vi "FipsAdjacent.vi"() -> (11 "Fips":i32[](array[numeric]))   [LabVIEW 2017] (continued)
\"Posey County, IN\"\t18129\n\"Posey County, IN\"\t18129\t\"Vanderburgh County, IN\"\t18163\n\"Posey County, IN\"\t18129\t\"Henderson County, KY\"\t21101\n\"Posey County, IN\"\t18129\t\"Union County, KY\"\t21225\n\"Pulaski County, IN\"\t18131\t\"Cass County, IN\"\t18017\n\"Pulaski County, IN\"\t18131\t\"Fulton County, IN\"\t18049\n\"Pulaski County, IN\"\t18131\t\"Jasper County, IN\"\t18073\n\"Pulaski County, IN\"\t18131\t\"Marshall County, IN\"\t18099\n\"Pulaski County, IN\"\t18131\t\"Pulaski County, IN\"\t18131\n\"Pulaski County, IN\"\t18131\t\"Starke County, IN\"\t18149\n\"Pulaski County, IN\"\t18131\t\"White County, IN\"\t18181\n\"Putnam County, IN\"\t18133\t\"Clay County, IN\"\t18021\n\"Putnam County, IN\"\t18133\t\"Hendricks County, IN\"\t18063\n\"Putnam County, IN\"\t18133\t\"Montgomery County, IN\"\t18107\n\"Putnam County, IN\"\t18133\t\"Morgan County, IN\"\t18109\n\"Putnam County, IN\"\t18133\t\"Owen County, IN\"\t18119\n\"Putnam County, IN\"\t18133\t\"Parke County, IN\"\t18121\n\"Putnam County, IN\"\t18133\t\"Putnam County, IN\"\t18133\n\"Randolph County, IN\"\t18135\t\"Delaware County, IN\"\t18035\n\"Randolph County, IN\"\t18135\t\"Henry County, IN\"\t18065\n\"Randolph County, IN\"\t18135\t\"Jay County, IN\"\t18075\n\"Randolph County, IN\"\t18135\t\"Randolph County, IN\"\t18135\n\"Randolph County, IN\"\t18135\t\"Wayne County, IN\"\t18177\n\"Randolph County, IN\"\t18135\t\"Darke County, OH\"\t39037\n\"Ripley County, IN\"\t18137\t\"Dearborn County, IN\"\t18029\n\"Ripley County, IN\"\t18137\t\"Decatur County, IN\"\t18031\n\"Ripley County, IN\"\t18137\t\"Franklin County, IN\"\t18047\n\"Ripley County, IN\"\t18137\t\"Jefferson County, IN\"\t18077\n\"Ripley County, IN\"\t18137\t\"Jennings County, IN\"\t18079\n\"Ripley County, IN\"\t18137\t\"Ohio County, IN\"\t18115\n\"Ripley County, IN\"\t18137\t\"Ripley County, IN\"\t18137\n\"Ripley County, IN\"\t18137\t\"Switzerland County, IN\"\t18155\n\"Rush County, IN\"\t18139\t\"Decatur County, IN\"\t18031\n\"Rush County, IN\"\t18139\t\"Fayette County, IN\"\t18041\n\"Rush County, IN\"\t18139\t\"Franklin County, IN\"\t18047\n\"Rush County, IN\"\t18139\t\"Hancock County, IN\"\t18059\n\"Rush County, IN\"\t18139\t\"Henry County, IN\"\t18065\n\"Rush County, IN\"\t18139\t\"Rush County, IN\"\t18139\n\"Rush County, IN\"\t18139\t\"Shelby County, IN\"\t18145\n\"St. Joseph County, IN\"\t18141\t\"Elkhart County, IN\"\t18039\n\"St. Joseph County, IN\"\t18141\t\"LaPorte County, IN\"\t18091\n\"St. Joseph County, IN\"\t18141\t\"Marshall County, IN\"\t18099\n\"St. Joseph County, IN\"\t18141\t\"St. Joseph County, IN\"\t18141\n\"St. Joseph County, IN\"\t18141\t\"Starke County, IN\"\t18149\n\"St. Joseph County, IN\"\t18141\t\"Berrien County, MI\"\t26021\n\"St. Joseph County, IN\"\t18141\t\"Cass County, MI\"\t26027\n\"Scott County, IN\"\t18143\t\"Clark County, IN\"\t18019\n\"Scott County, IN\"\t18143\t\"Jackson County, IN\"\t18071\n\"Scott County, IN\"\t18143\t\"Jefferson County, IN\"\t18077\n\"Scott County, IN\"\t18143\t\"Jennings County, IN\"\t18079\n\"Scott County, IN\"\t18143\t\"Scott County, IN\"\t18143\n\"Scott County, IN\"\t18143\t\"Washington County, IN\"\t18175\n\"Shelby County, IN\"\t18145\t\"Bartholomew County, IN\"\t18005\n\"Shelby County, IN\"\t18145\t\"Decatur County, IN\"\t18031\n\"Shelby County, IN\"\t18145\t\"Hancock County, IN\"\t18059\n\"Shelby County, IN\"\t18145\t\"Johnson County, IN\"\t18081\n\"Shelby County, IN\"\t18145\t\"Marion County, IN\"\t18097\n\"Shelby County, IN\"\t18145\t\"Rush County, IN\"\t18139\n\"Shelby County, IN\"\t18145\t\"Shelby County, IN\"\t18145\n\"Spencer County, IN\"\t18147\t\"Dubois County, IN\"\t18037\n\"Spencer County, IN\"\t18147\t\"Perry County, IN\"\t18123\n\"Spencer County, IN\"\t18147\t\"Spencer County, IN\"\t18147\n\"Spencer County, IN\"\t18147\t\"Warrick County, IN\"\t18173\n\"Spencer County, IN\"\t18147\t\"Daviess County, KY\"\t21059\n\"Spencer County, IN\"\t18147\t\"Hancock County, KY\"\t21091\n\"Starke County, IN\"\t18149\t\"Fulton County, IN\"\t18049\n\"Starke County, IN\"\t18149\t\"Jasper County, IN\"\t18073\n\"Starke County, IN\"\t18149\t\"LaPorte County, IN\"\t18091\n\"Starke County, IN\"\t18149\t\"Marshall County, IN\"\t18099\n\"Starke County, IN\"\t18149\t\"Porter County, IN\"\t18127\n\"Starke County, IN\"\t18149\t\"Pulaski County, IN\"\t18131\n\"Starke County, IN\"\t18149\t\"St. Joseph County, IN\"\t18141\n\"Starke County, IN\"\t18149\t\"Starke County, IN\"\t18149\n\"Steuben County, IN\"\t18151\t\"DeKalb County, IN\"\t18033\n\"Steuben County, IN\"\t18151\t\"LaGrange County, IN\"\t18087\n\"Steuben County, IN\"\t18151\t\"Noble County, IN\"\t18113\n\"Steuben County, IN\"\t18151\t\"Steuben County, IN\"\t18151\n\"Steuben County, IN\"\t18151\t\"Branch County, MI\"\t26023\n\"Steuben County, IN\"\t18151\t\"Hillsdale County, MI\"\t26059\n\"Steuben County, IN\"\t18151\t\"Williams County, OH\"\t39171\n\"Sullivan County, IN\"\t18153\t\"Clark County, IL\"\t17023\n\"Sullivan County, IN\"\t18153\t\"Crawford County, IL\"\t17033\n\"Sullivan County, IN\"\t18153\t\"Clay County, IN\"\t18021\n\"Sullivan County, IN\"\t18153\t\"Greene County, IN\"\t18055\n\"Sullivan County, IN\"\t18153\t\"Knox County, IN\"\t18083\n\"Sullivan County, IN\"\t18153\t\"Sullivan County, IN\"\t18153\n\"Sullivan County, IN\"\t18153\t\"Vigo County, IN\"\t18167\n\"Switzerland County, IN\"\t18155\t\"Jefferson County, IN\"\t18077\n\"Switzerland County, IN\"\t18155\t\"Ohio County, IN\"\t18115\n\"Switzerland County, IN\"\t18155\t\"Ripley County, IN\"\t18137\n\"Switzerland County, IN\"\t18155\t\"Switzerland County, IN\"\t18155\n\"Switzerland County, IN\"\t18155\t\"Boone County, KY\"\t21015\n\"Switzerland County, IN\"\t18155\t\"Carroll County, KY\"\t21041\n\"Switzerland County, IN\"\t18155\t\"Gallatin County, KY\"\t21077\n\"Tippecanoe County, IN\"\t18157\t\"Benton County, IN\"\t18007\n\"Tippecanoe County, IN\"\t18157\t\"Carroll County, IN\"\t18015\n\"Tippecanoe County, IN\"\t18157\t\"Clinton County, IN\"\t18023\n\"Tippecanoe County, IN\"\t18157\t\"Fountain County, IN\"\t18045\n\"Tippecanoe County, IN\"\t18157\t\"Montgomery County, IN\"\t18107\n\"Tippecanoe County, IN\"\t18157\t\"Tippecanoe County, IN\"\t18157\n\"Tippecanoe County, IN\"\t18157\t\"Warren County, IN\"\t18171\n\"Tippecanoe County, IN\"\t18157\t\"White County, IN\"\t18181\n\"Tipton County, IN\"\t18159\t\"Clinton County, IN\"\t18023\n\"Tipton County, IN\"\t18159\t\"Grant County, IN\"\t18053\n\"Tipton County, IN\"\t18159\t\"Hamilton County, IN\"\t18057\n\"Tipton County, IN\"\t18159\t\"Howard County, IN\"\t18067\n\"Tipton County, IN\"\t18159\t\"Madison County, IN\"\t18095\n\"Tipton County, IN\"\t18159\t\"Tipton County, IN\"\t18159\n\"Union County, IN\"\t18161\t\"Fayette County, IN\"\t18041\n\"Union County, IN\"\t18161\t\"Franklin County, IN\"\t18047\n\"Union County, IN\"\t18161\t\"Union County, IN\"\t18161\n\"Union County, IN\"\t18161\t\"Wayne County, IN\"\t18177\n\"Union County, IN\"\t18161\t\"Butler County, OH\"\t39017\n\"Union County, IN\"\t18161\t\"Preble County, OH\"\t39135\n\"Vanderburgh County, IN\"\t18163\t\"Gibson County, IN\"\t18051\n\"Vanderburgh County, IN\"\t18163\t\"Posey County, IN\"\t18129\n\"Vanderburgh County, IN\"\t18163\t\"Vanderburgh County, IN\"\t18163\n\"Vanderburgh County, IN\"\t18163\t\"Warrick County, IN\"\t18173\n\"Vanderburgh County, IN\"\t18163\t\"Henderson County, KY\"\t21101\n\"Vermillion County, IN\"\t18165\t\"Edgar County, IL\"\t17045\n\"Vermillion County, IN\"\t18165\t\"Vermilion County, IL\"\t17183\n\"Vermillion County, IN\"\t18165\t\"Fountain County, IN\"\t18045\n\"Vermillion County, IN\"\t18165\t\"Parke County, IN\"\t18121\n\"Vermillion County, IN\"\t18165\t\"Vermillion County, IN\"\t18165\n\"Vermillion County, IN\"\t18165\t\"Vigo County, IN\"\t18167\n\"Vermillion County, IN\"\t18165\t\"Warren County, IN\"\t18171\n\"Vigo County, IN\"\t18167\t\"Clark County, IL\"\t17023\n\"Vigo County, IN\"\t18167\t\"Edgar County, IL\"\t17045\n\"Vigo County, IN\"\t18167\t\"Clay County, IN\"\t18021\n\"Vigo County, IN\"\t18167\t\"Parke County, IN\"\t18121\n\"Vigo County, IN\"\t18167\t\"Sullivan County, IN\"\t18153\n\"Vigo County, IN\"\t18167\t\"Vermillion County, IN\"\t18165\n\"Vigo County, IN\"\t18167\t\"Vigo County, IN\"\t18167\n\"Wabash County, IN\"\t18169\t\"Fulton County, IN\"\t18049\n\"Wabash County, IN\"\t18169\t\"Grant County, IN\"\t18053\n\"Wabash County, IN\"\t18169\t\"Huntington County, IN\"\t18069\n\"Wabash County, IN\"\t18169\t\"Kosciusko County, IN\"\t18085\n\"Wabash County, IN\"\t18169\t\"Miami County, IN\"\t18103\n\"Wabash County, IN\"\t18169\t\"Wabash County, IN\"\t18169\n\"Wabash County, IN\"\t18169\t\"Whitley County, IN\"\t18183\n\"Warren County, IN\"\t18171\t\"Vermilion County, IL\"\t17183\n\"Warren County, IN\"\t18171\t\"Benton County, IN\"\t18007\n\"Warren County, IN\"\t18171\t\"Fountain County, IN\"\t18045\n\"Warren County, IN\"\t18171\t\"Tippecanoe County, IN\"\t18157\n\"Warren County, IN\"\t18171\t\"Vermillion County, IN\"\t18165\n\"Warren County, IN\"\t18171\t\"Warren County, IN\"\t18171\n\"Warrick County, IN\"\t18173\t\"Dubois County, IN\"\t18037\n\"Warrick County, IN\"\t18173\t\"Gibson County, IN\"\t18051\n\"Warrick County, IN\"\t18173\t\"Pike County, IN\"\t18125\n\"Warrick County, IN\"\t18173\t\"Spencer County, IN\"\t18147\n\"Warrick County, IN\"\t18173\t\"Vanderburgh County, IN\"\t18163\n\"Warrick County, IN\"\t18173\t\"Warrick County, IN\"\t18173\n\"Warrick County, IN\"\t18173\t\"Daviess County, KY\"\t21059\n\"Warrick County, IN\"\t18173\t\"Henderson County, KY\"\t21101\n\"Washington County, IN\"\t18175\t\"Clark County, IN\"\t18019\n\"Washington County, IN\"\t18175\t\"Crawford County, IN\"\t18025\n\"Washington County, IN\"\t18175\t\"Floyd County, IN\"\t18043\n\"Washington County, IN\"\t18175\t\"Harrison County, IN\"\t18061\n\"Washington County, IN\"\t18175\t\"Jackson County, IN\"\t18071\n\"Washington County, IN\"\t18175\t\"Lawrence County, IN\"\t18093\n\"Washington County, IN\"\t18175\t\"Orange County, IN\"\t18117\n\"Washington County, IN\"\t18175\t\"Scott County, IN\"\t18143\n\"Washington County, IN\"\t18175\t\"Washington County, IN\"\t18175\n\"Wayne County, IN\"\t18177\t\"Fayette County, IN\"\t18041\n\"Wayne County, IN\"\t18177\t\"Henry County, IN\"\t18065\n\"Wayne County, IN\"\t18177\t\"Randolph County, IN\"\t18135\n\"Wayne County, IN\"\t18177\t\"Union County, IN\"\t18161\n\"Wayne County, IN\"\t18177\t\"Wayne County, IN\"\t18177\n\"Wayne County, IN\"\t18177\t\"Darke County, OH\"\t39037\n\"Wayne County, IN\"\t18177\t\"Preble County, OH\"\t39135\n\"Wells County, IN\"\t18179\t\"Adams County, IN\"\t18001\n\"Wells County, IN\"\t18179\t\"Allen County, IN\"\t18003\n\"Wells County, IN\"\t18179\t\"Blackford County, IN\"\t18009\n\"Wells County, IN\"\t18179\t\"Grant County, IN\"\t18053\n\"Wells County, IN\"\t18179\t\"Huntington County, IN\"\t18069\n\"Wells County, IN\"\t18179\t\"Jay County, IN\"\t18075\n\"Wells County, IN\"\t18179\t\"Wells County, IN\"\t18179\n\"White County, IN\"\t18181\t\"Benton County, IN\"\t18007\n\"White County, IN\"\t18181\t\"Carroll County, IN\"\t18015\n\"White County, IN\"\t18181\t\"Cass County, IN\"\t18017\n\"White County, IN\"\t18181\t\"Jasper County, IN\"\t18073\n\"White County, IN\"\t18181\t\"Pulaski County, IN\"\t18131\n\"White County, IN\"\t18181\t\"Tippecanoe County, IN\"\t18157\n\"White County, IN\"\t18181\t\"White County, IN\"\t18181\n\"Whitley County, IN\"\t18183\t\"Allen County, IN\"\t18003\n\"Whitley County, IN\"\t18183\t\"Huntington County, IN\"\t18069\n\"Whitley County, IN\"\t18183\t\"Kosciusko County, IN\"\t18085\n\"Whitley County, IN\"\t18183\t\"Noble County, IN\"\t18113\n\"Whitley County, IN\"\t18183\t\"Wabash County, IN\"\t18169\n\"Whitley County, IN\"\t18183\t\"Whitley County, IN\"\t18183\n\"Adair County, IA\"\t19001\t\"Adair County, IA\"\t19001\n\"Adair County, IA\"\t19001\t\"Adams County, IA\"\t19003\n\"Adair County, IA\"\t19001\t\"Audubon County, IA\"\t19009\n\"Adair County, IA\"\t19001\t\"Cass County, IA\"\t19029\n\"Adair County, IA\"\t19001\t\"Dallas County, IA\"\t19049\n\"Adair County, IA\"\t19001\t\"Guthrie County, IA\"\t19077\n\"Adair County, IA\"\t19001\t\"Madison County, IA\"\t19121\n\"Adair County, IA\"\t19001\t\"Union County, IA\"\t19175\n\"Adams County, IA\"\t19003\t\"Adair County, IA\"\t19001\n\"Adams County, IA\"\t19003\t\"Adams County, IA\"\t19003\n\"Adams County, IA\"\t19003\t\"Cass County, IA\"\t19029\n\"Adams County, IA\"\t19003\t\"Montgomery County, IA\"\t19137\n\"Adams County, IA\"\t19003\t\"Page County, IA\"\t19145\n\"Adams County, IA\"\t19003\t\"Ringgold County, IA\"\t19159\n\"Adams County, IA\"\t19003\t\"Taylor County, IA\"\t19173\n\"Adams County, IA\"\t19003\t\"Union County, IA\"\t19175\n\"Allamakee County, IA\"\t19005\t\"Allamakee County, IA\"\t19005\n\"Allamakee County, IA\"\t19005\t\"Clayton County, IA\"\t19043\n\"Allamakee County, IA\"\t19005\t\"Fayette County, IA\"\t19065\n\"Allamakee County, IA\"\t19005\t\"Winneshiek County, IA\"\t19191\n\"Allamakee County, IA\"\t19005\t\"Houston County, MN\"\t27055\n\"Allamakee County, IA\"\t19005\t\"Crawford County, WI\"\t55023\n\"Allamakee County, IA\"\t19005\t\"Vernon County, WI\"\t55123\n\"Appanoose County, IA\"\t19007\t\"Appanoose County, IA\"\t19007\n\"Appanoose County, IA\"\t19007\t\"Davis County, IA\"\t19051\n\"Appanoose County, IA\"\t19007\t\"Lucas County, IA\"\t19117\n\"Appanoose County, IA\"\t19007\t\"Monroe County, IA\"\t19135\n\"Appanoose County, IA\"\t19007\t\"Wapello County, IA\"\t19179\n\"Appanoose County, IA\"\t19007\t\"Wayne County, IA\"\t19185\n\"Appanoose County, IA\"\t19007\t\"Putnam County, MO\"\t29171\n\"Appanoose County, IA\"\t19007\t\"Schuyler County, MO\"\t29197\n\"Audubon County, IA\"\t19009\t\"Adair County, IA\"\t19001\n\"Audubon County, IA\"\t19009\t\"Audubon County, IA\"\t19009\n\"Audubon County, IA\"\t19009\t\"Carroll County, IA\"\t19027\n\"Audubon County, IA\"\t19009\t\"Cass County, IA\"\t19029\n\"Audubon County, IA\"\t19009\t\"Crawford County, IA\"\t19047\n\"Audubon County, IA\"\t19009\t\"Guthrie County, IA\"\t19077\n\"Audubon County, IA\"\t19009\t\"Shelby County, IA\"\t19165\n\"Benton County, IA\"\t19011\t\"Benton County, IA\"\t19011\n\"Benton County, IA\"\t19011\t\"Black Hawk County, IA\"\t19013\n\"Benton County, IA\"\t19011\t\"Buchanan County, IA\"\t19019\n\"Benton County, IA\"\t19011\t\"Iowa County, IA\"\t19095\n\"Benton County, IA\"\t19011\t\"Johnson County, IA\"\t19103\n\"Benton County, IA\"\t19011\t\"Linn County, IA\"\t19113\n\"Benton County, IA\"\t19011\t\"Poweshiek County, IA\"\t19157\n\"Benton County, IA\"\t19011\t\"Tama County, IA\"\t19171\n\"Black Hawk County, IA\"\t19013\t\"Benton County, IA\"\t19011\n\"Black Hawk County, IA\"\t19013\t\"Black Hawk County, IA\"\t19013\n\"Black Hawk County, IA\"\t19013\t\"Bremer County, IA\"\t19017\n\"Black Hawk County, IA\"\t19013\t\"Buchanan County, IA\"\t19019\n\"Black Hawk County, IA\"\t19013\t\"Butler County, IA\"\t19023\n\"Black Hawk County, IA\"\t19013\t\"Fayette County, IA\"\t19065\n\"Black Hawk County, IA\"\t19013\t\"Grundy County, IA\"\t19075\n\"Black Hawk County, IA\"\t19013\t\"Tama County, IA\"\t19171\n\"Boone County, IA\"\t19015\t\"Boone County, IA\"\t19015\n\"Boone County, IA\"\t19015\t\"Dallas County, IA\"\t19049\n\"Boone County, IA\"\t19015\t\"Greene County, IA\"\t19073\n\"Boone County, IA\"\t19015\t\"Hamilton County, IA\"\t19079\n\"Boone County, IA\"\t19015\t\"Polk County, IA\"\t19153\n\"Boone County, IA\"\t19015\t\"Story County, IA\"\t19169\n\"Boone County, IA\"\t19015\t\"Webster County, IA\"\t19187\n\"Bremer County, IA\"\t19017\t\"Black Hawk County, IA\"\t19013\n\"Bremer County, IA\"\t19017\t\"Bremer County, IA\"\t19017\n\"Bremer County, IA\"\t19017\t\"Buchanan County, IA\"\t19019\n\"Bremer County, IA\"\t19017\t\"Butler County, IA\"\t19023\n\"Bremer County, IA\"\t19017\t\"Chickasaw County, IA\"\t19037\n\"Bremer County, IA\"\t19017\t\"Fayette County, IA\"\t19065\n\"Bremer County, IA\"\t19017\t\"Floyd County, IA\"\t19067\n\"Buchanan County, IA\"\t19019\t\"Benton County, IA\"\t19011\n\"Buchanan County, IA\"\t19019\t\"Black Hawk County, IA\"\t19013\n\"Buchanan County, IA\"\t19019\t\"Bremer County, IA\"\t19017\n\"Buchanan County, IA\"\t19019\t\"Buchanan County, IA\"\t19019\n\"Buchanan County, IA\"\t19019\t\"Clayton County, IA\"\t19043\n\"Buchanan County, IA\"\t19019\t\"Delaware County, IA\"\t19055\n\"Buchanan County, IA\"\t19019\t\"Fayette County, IA\"\t19065\n\"Buchanan County, IA\"\t19019\t\"Linn County, IA\"\t19113\n\"Buena Vista County, IA\"\t19021\t\"Buena Vista County, IA\"\t19021\n\"Buena Vista County, IA\"\t19021\t\"Calhoun County, IA\"\t19025\n\"Buena Vista County, IA\"\t19021\t\"Cherokee County, IA\"\t19035\n\"Buena Vista County, IA\"\t19021\t\"Clay County, IA\"\t19041\n\"Buena Vista County, IA\"\t19021\t\"Ida County, IA\"\t19093\n\"Buena Vista County, IA\"\t19021\t\"O'Brien County, IA\"\t19141\n\"Buena Vista County, IA\"\t19021\t\"Palo Alto County, IA\"\t19147\n\"Buena Vista County, IA\"\t19021\t\"Pocahontas County, IA\"\t19151\n\"Buena Vista County, IA\"\t19021\t\"Sac County, IA\"\t19161\n\"Butler County, IA\"\t19023\t\"Black Hawk County, IA\"\t19013\n\"Butler County, IA\"\t19023\t\"Bremer County, IA\"\t19017\n\"Butler County, IA\"\t19023\t\"Butler County, IA\"\t19023\n\"Butler County, IA\"\t19023\t\"Cerro Gordo County, IA\"\t19033\n\"Butler County, IA\"\t19023\t\"Chickasaw County, IA\"\t19037\n\"Butler County, IA\"\t19023\t\"Floyd County, IA\"\t19067\n\"Butler County, IA\"\t19023\t\"Franklin County, IA\"\t19069\n\"Butler County, IA\"\t19023\t\"Grundy County, IA\"\t19075\n\"Butler County, IA\"\t19023\t\"Hardin County, IA\"\t19083\n\"Calhoun County, IA\"\t19025\t\"Buena Vista County, IA\"\t19021\n\"Calhoun County, IA\"\t19025\t\"Calhoun County, IA\"\t19025\n\"Calhoun County, IA\"\t19025\t\"Carroll County, IA\"\t19027\n\"Calhoun County, IA\"\t19025\t\"Greene County, IA\"\t19073\n\"Calhoun County, IA\"\t19025\t\"Pocahontas County, IA\"\t19151\n\"Calhoun County, IA\"\t19025\t\"Sac County, IA\"\t19161\n\"Calhoun County, IA\"\t19025\t\"Webster County, IA\"\t19187\n\"Carroll County, IA\"\t19027\t\"Audubon County, IA\"\t19009\n\"Carroll County, IA\"\t19027\t\"Calhoun County, IA\"\t19025\n\"Carroll County, IA\"\t19027\t\"Carroll County, IA\"\t19027\n\"Carroll County, IA\"\t19027\t\"Crawford County, IA\"\t19047\n\"Carroll County, IA\"\t19027\t\"Greene County, IA\"\t19073\n\"Carroll County, IA\"\t19027\t\"Guthrie County, IA\"\t19077\n\"Carroll County, IA\"\t19027\t\"Sac County, IA\"\t19161\n\"Carroll County, IA\"\t19027\t\"Shelby County, IA\"\t19165\n\"Cass County, IA\"\t19029\t\"Adair County, IA\"\t19001\n\"Cass County, IA\"\t19029\t\"Adams County, IA\"\t19003\n\"Cass County, IA\"\t19029\t\"Audubon County, IA\"\t19009\n\"Cass County, IA\"\t19029\t\"Cass County, IA\"\t19029\n\"Cass County, IA\"\t19029\t\"Guthrie County, IA\"\t19077\n\"Cass County, IA\"\t19029\t\"Montgomery County, IA\"\t19137\n\"Cass County, IA\"\t19029\t\"Pottawattamie County, IA\"\t19155\n\"Cass County, IA\"\t19029\t\"Shelby County, IA\"\t19165\n\"Cedar County, IA\"\t19031\t\"Cedar County, IA\"\t19031\n\"Cedar County, IA\"\t19031\t\"Clinton County, IA\"\t19045\n\"Cedar County, IA\"\t19031\t\"Johnson County, IA\"\t19103\n\"Cedar County, IA\"\t19031\t\"Jones County, IA\"\t19105\n\"Cedar County, IA\"\t19031\t\"Linn County, IA\"\t19113\n\"Cedar County, IA\"\t19031\t\"Muscatine County, IA\"\t19139\n\"Cedar County, IA\"\t19031\t\"Scott County, IA\"\t19163\n\"Cerro Gordo County, IA\"\t19033\t\"Butler County, IA\"\t19023\n\"Cerro Gordo County, IA\"\t19033\t\"Cerro Gordo County, IA\"\t19033\n\"Cerro Gordo County, IA\"\t19033\t\"Floyd County, IA\"\t19067\n\"Cerro Gordo County, IA\"\t19033\t\"Franklin County, IA\"\t19069\n\"Cerro Gordo County, IA\"\t19033\t\"Hancock County, IA\"\t19081\n\"Cerro Gordo County, IA\"\t19033\t\"Mitchell County, IA\"\t19131\n\"Cerro Gordo County, IA\"\t19033\t\"Winnebago County, IA\"\t19189\n\"Cerro Gordo County, IA\"\t19033\t\"Worth County, IA\"\t19195\n\"Cerro Gordo County, IA\"\t19033\t\"Wright County, IA\"\t19197\n\"Cherokee County, IA\"\t19035\t\"Buena Vista County, IA\"\t19021\n\"Cherokee County, IA\"\t19035\t\"Cherokee County, IA\"\t19035\n\"Cherokee County, IA\"\t19035\t\"Clay County, IA\"\t19041\n\"Cherokee County, IA\"\t19035\t\"Ida County, IA\"\t19093\n\"Cherokee County, IA\"\t19035\t\"O'Brien County, IA\"\t19141\n\"Cherokee County, IA\"\t19035\t\"Plymouth County, IA\"\t19149\n\"Cherokee County, IA\"\t19035\t\"Sac County, IA\"\t19161\n\"Cherokee County, IA\"\t19035\t\"Sioux County, IA\"\t19167\n\"Cherokee County, IA\"\t19035\t\"Woodbury County, IA\"\t19193\n\"Chickasaw County, IA\"\t19037\t\"Bremer County, IA\"\t19017\n\"Chickasaw County, IA\"\t19037\t\"Butler County, IA\"\t19023\n\"Chickasaw County, IA\"\t19037\t\"Chickasaw County, IA\"\t19037\n\"Chickasaw County, IA\"\t19037\t\"Fayette County, IA\"\t19065\n\"Chickasaw County, IA\"\t19037\t\"Floyd County, IA\"\t19067\n\"Chickasaw County, IA\"\t19037\t\"Howard County, IA\"\t19089\n\"Chickasaw County, IA\"\t19037\t\"Mitchell County, IA\"\t19131\n\"Chickasaw County, IA\"\t19037\t\"Winneshiek County, IA\"\t19191\n\"Clarke County, IA\"\t19039\t\"Clarke County, IA\"\t19039\n\"Clarke County, IA\"\t19039\t\"Decatur County, IA\"\t19053\n\"Clarke County, IA\"\t19039\t\"Lucas County, IA\"\t19117\n\"Clarke County, IA\"\t19039\t\"Madison County, IA\"\t19121\n\"Clarke County, IA\"\t19039\t\"Ringgold County, IA\"\t19159\n\"Clarke County, IA\"\t19039\t\"Union County, IA\"\t19175\n\"Clarke County, IA\"\t19039\t\"Warren County, IA\"\t19181\n\"Clarke County, IA\"\t19039\t\"Wayne County, IA\"\t19185\n\"Clay County, IA\"\t19041\t\"Buena Vista County, IA\"\t19021\n\"Clay County, IA\"\t19041\t\"Cherokee County, IA\"\t19035\n\"Clay County, IA\"\t19041\t\"Clay County, IA\"\t19041\n\"Clay County, IA\"\t19041\t\"Dickinson County, IA\"\t19059\n\"Clay County, IA\"\t19041\t\"Emmet County, IA\"\t19063\n\"Clay County, IA\"\t19041\t\"O'Brien County, IA\"\t19141\n\"Clay County, IA\"\t19041\t\"Osceola County, IA\"\t19143\n\"Clay County, IA\"\t19041\t\"Palo Alto County, IA\"\t19147\n\"Clay County, IA\"\t19041\t\"Pocahontas County, IA\"\t19151\n\"Clayton County, IA\"\t19043\t\"Allamakee County, IA\"\t19005\n\"Clayton County, IA\"\t19043\t\"Buchanan County, IA\"\t19019\n\"Clayton County, IA\"\t19043\t\"Clayton County, IA\"\t19043\n\"Clayton County, IA\"\t19043\t\"Delaware County, IA\"\t19055\n\"Clayton County, IA\"\t19043\t\"Dubuque County, IA\"\t19061\n\"Clayton County, IA\"\t19043\t\"Fayette County, IA\"\t19065\n\"Clayton County, IA\"\t19043\t\"Winneshiek County, IA\"\t19191\n\"Clayton County, IA\"\t19043\t\"Crawford County, WI\"\t55023\n\"Clayton County, IA\"\t19043\t\"Grant County, WI\"\t55043\n\"Clinton County, IA\"\t19045\t\"Carroll County, IL\"\t17015\n\"Clinton County, IA\"\t19045\t\"Rock Island County, IL\"\t17161\n\"Clinton County, IA\"\t19045\t\"Whiteside County, IL\"\t17195\n\"Clinton County, IA\"\t19045\t\"Cedar County, IA\"\t19031\n\"Clinton County, IA\"\t19045\t\"Clinton County, IA\"\t19045\n\"Clinton County, IA\"\t19045\t\"Jackson County, IA\"\t19097\n\"Clinton County, IA\"\t19045\t\"Jones County, IA\"\t19105\n\"Clinton County, IA\"\t19045\t\"Scott County, IA\"\t19163\n\"Crawford County, IA\"\t19047\t\"Audubon County, IA\"\t19009\n\"Crawford County, IA\"\t19047\t\"Carroll County, IA\"\t19027\n\"Crawford County, IA\"\t19047\t\"Crawford County, IA\"\t19047\n\"Crawford County, IA\"\t19047\t\"Harrison County, IA\"\t19085\n\"Crawford County, IA\"\t19047\t\"Ida County, IA\"\t19093\n\"Crawford County, IA\"\t19047\t\"Monona County, IA\"\t19133\n\"Crawford County, IA\"\t19047\t\"Sac County, IA\"\t19161\n\"Crawford County, IA\"\t19047\t\"Shelby County, IA\"\t19165\n\"Crawford County, IA\"\t19047\t\"Woodbury County, IA\"\t19193\n\"Dallas County, IA\"\t19049\t\"Adair County, IA\"\t19001\n\"Dallas County, IA\"\t19049\t\"Boone County, IA\"\t19015\n\"Dallas County, IA\"\t19049\t\"Dallas County, IA\"\t19049\n\"Dallas County, IA\"\t19049\t\"Greene County, IA\"\t19073\n\"Dallas County, IA\"\t19049\t\"Guthrie County, IA\"\t19077\n\"Dallas County, IA\"\t19049\t\"Madison County, IA\"\t19121\n\"Dallas County, IA\"\t19049\t\"Polk County, IA\"\t19153\n\"Dallas County, IA\"\t19049\t\"Warren County, IA\"\t19181\n\"Davis County, IA\"\t19051\t\"Appanoose County, IA\"\t19007\n\"Davis County, IA\"\t19051\t\"Davis County, IA\"\t19051\n\"Davis County, IA\"\t19051\t\"Jefferson County, IA\"\t19101\n\"Davis County, IA\"\t19051\t\"Monroe County, IA\"\t19135\n\"Davis County, IA\"\t19051\t\"Van Buren County, IA\"\t19177\n\"Davis County, IA\"\t19051\t\"Wapello County, IA\"\t19179\n\"Davis County, IA\"\t19051\t\"Schuyler County, MO\"\t29197\n\"Davis County, IA\"\t19051\t\"Scotland County, MO\"\t29199\n\"Decatur County, IA\"\t19053\t\"Clarke County, IA\"\t19039\n\"Decatur County, IA\"\t19053\t\"Decatur County, IA\"\t19053\n\"Decatur County, IA\"\t19053\t\"Lucas County, IA\"\t19117\n\"Decatur County, IA\"\t19053\t\"Ringgold County, IA\"\t19159\n\"Decatur County, IA\"\t19053\t\"Union County, IA\"\t19175\n\"Decatur County, IA\"\t19053\t\"Wayne County, IA\"\t19185\n\"Decatur County, IA\"\t19053\t\"Harrison County, MO\"\t29081\n\"Decatur County, IA\"\t19053\t\"Mercer County, MO\"\t29129\n\"Delaware County, IA\"\t19055\t\"Buchanan County, IA\"\t19019\n\"Delaware County, IA\"\t19055\t\"Clayton County, IA\"\t19043\n\"Delaware County, IA\"\t19055\t\"Delaware County, IA\"\t19055\n\"Delaware County, IA\"\t19055\t\"Dubuque County, IA\"\t19061\n\"Delaware County, IA\"\t19055\t\"Fayette County, IA\"\t19065\n\"Delaware County, IA\"\t19055\t\"Jones County, IA\"\t19105\n\"Delaware County, IA\"\t19055\t\"Linn County, IA\"\t19113\n\"Des Moines County, IA\"\t19057\t\"Henderson County, IL\"\t17071\n\"Des Moines County, IA\"\t19057\t\"Mercer County, IL\"\t17131\n\"Des Moines County, IA\"\t19057\t\"Des Moines County, IA\"\t19057\n\"Des Moines County, IA\"\t19057\t\"Henry County, IA\"\t19087\n\"Des Moines County, IA\"\t19057\t\"Lee County, IA\"\t19111\n\"Des Moines County, IA\"\t19057\t\"Louisa County, IA\"\t19115\n\"Dickinson County, IA\"\t19059\t\"Clay County, IA\"\t19041\n\"Dickinson County, IA\"\t19059\t\"Dickinson County, IA\"\t19059\n\"Dickinson County, IA\"\t19059\t\"Emmet County, IA\"\t19063\n\"Dickinson County, IA\"\t19059\t\"O'Brien County, IA\"\t19141\n\"Dickinson County, IA\"\t19059\t\"Osceola County, IA\"\t19143\n\"Dickinson County, IA\"\t19059\t\"Palo Alto County, IA\"\t19147\n\"Dickinson County, IA\"\t19059\t\"Jackson County, MN\"\t27063\n\"Dubuque County, IA\"\t19061\t\"Jo Daviess County, IL\"\t17085\n\"Dubuque County, IA\"\t19061\t\"Clayton County, IA\"\t19043\n\"Dubuque County, IA\"\t19061\t\"Delaware County, IA\"\t19055\n\"Dubuque County, IA\"\t19061\t\"Dubuque County, IA\"\t19061\n\"Dubuque County, IA\"\t19061\t\"Jackson County, IA\"\t19097\n\"Dubuque County, IA\"\t19061\t\"Jones County, IA\"\t19105\n\"Dubuque County, IA\"\t19061\t\"Grant County, WI\"\t55043\n\"Emmet County, IA\"\t19063\t\"Clay County, IA\"\t19041\n\"Emmet County, IA\"\t19063\t\"Dickinson County, IA\"\t19059\n\"Emmet County, IA\"\t19063\t\"Emmet County, IA\"\t19063\n\"Emmet County, IA\"\t19063\t\"Kossuth County, IA\"\t19109\n\"Emmet County, IA\"\t19063\t\"Palo Alto County, IA\"\t19147\n\"Emmet County, IA\"\t19063\t\"Jackson County, MN\"\t27063\n\"Emmet County, IA\"\t19063\t\"Martin County, MN\"\t27091\n\"Fayette County, IA\"\t19065\t\"Allamakee County, IA\"\t19005\n\"Fayette County, IA\"\t19065\t\"Black Hawk County, IA\"\t19013\n\"Fayette County, IA\"\t19065\t\"Bremer County, IA\"\t19017\n\"Fayette County, IA\"\t19065\t\"Buchanan County, IA\"\t19019\n\"Fayette County, IA\"\t19065\t\"Chickasaw County, IA\"\t19037\n\"Fayette County, IA\"\t19065\t\"Clayton County, IA\"\t19043\n\"Fayette County, IA\"\t19065\t\"Delaware County, IA\"\t19055\n\"Fayette County, IA\"\t19065\t\"Fayette County, IA\"\t19065\n\"Fayette County, IA\"\t19065\t\"Winneshiek County, IA\"\t19191\n\"Floyd County, IA\"\t19067\t\"Bremer County, IA\"\t19017\n\"Floyd County, IA\"\t19067\t\"Butler County, IA\"\t19023\n\"Floyd County, IA\"\t19067\t\"Cerro Gordo County, IA\"\t19033\n\"Floyd County, IA\"\t19067\t\"Chickasaw County, IA\"\t19037\n\"Floyd County, IA\"\t19067\t\"Floyd County, IA\"\t19067\n\"Floyd County, IA\"\t19067\t\"Franklin County, IA\"\t19069\n\"Floyd County, IA\"\t19067\t\"Howard County, IA\"\t19089\n\"Floyd County, IA\"\t19067\t\"Mitchell County, IA\"\t19131\n\"Franklin County, IA\"\t19069\t\"Butler County, IA\"\t19023\n\"Franklin County, IA\"\t19069\t\"Cerro Gordo County, IA\"\t19033\n\"Franklin County, IA\"\t19069\t\"Floyd County, IA\"\t19067\n\"Franklin County, IA\"\t19069\t\"Franklin County, IA\"\t19069\n\"Franklin County, IA\"\t19069\t\"Grundy County, IA\"\t19075\n\"Franklin County, IA\"\t19069\t\"Hamilton County, IA\"\t19079\n\"Franklin County, IA\"\t19069\t\"Hancock County, IA\"\t19081\n\"Franklin County, IA\"\t19069\t\"Hardin County, IA\"\t19083\n\"Franklin County, IA\"\t19069\t\"Wright County, IA\"\t19197\n\"Fremont County, IA\"\t19071\t\"Fremont County, IA\"\t19071\n\"Fremont County, IA\"\t19071\t\"Mills County, IA\"\t19129\n\"Fremont County, IA\"\t19071\t\"Montgomery County, IA\"\t19137\n\"Fremont County, IA\"\t19071\t\"Page County, IA\"\t19145\n\"Fremont County, IA\"\t19071\t\"Atchison County, MO\"\t29005\n\"Fremont County, IA\"\t19071\t\"Cass County, NE\"\t31025\n\"Fremont County, IA\"\t19071\t\"Otoe County, NE\"\t31131\n\"Greene County, IA\"\t19073\t\"Boone County, IA\"\t19015\n\"Greene County, IA\"\t19073\t\"Calhoun County, IA\"\t19025\n\"Greene County, IA\"\t19073\t\"Carroll County, IA\"\t19027\n\"Greene County, IA\"\t19073\t\"Dallas County, IA\"\t19049\n\"Greene County, IA\"\t19073\t\"Greene County, IA\"\t19073\n\"Greene County, IA\"\t19073\t\"Guthrie County, IA\"\t19077\n\"Greene County, IA\"\t19073\t\"Webster County, IA\"\t19187\n\"Grundy County, IA\"\t19075\t\"Black Hawk County, IA\"\t19013\n\"Grundy County, IA\"\t19075\t\"Butler County, IA\"\t19023\n\"Grundy County, IA\"\t19075\t\"Franklin County, IA\"\t19069\n\"Grundy County, IA\"\t19075\t\"Grundy County, IA\"\t19075\n\"Grundy County, IA\"\t19075\t\"Hardin County, IA\"\t19083\n\"Grundy County, IA\"\t19075\t\"Marshall County, IA\"\t19127\n\"Grundy County, IA\"\t19075\t\"Tama County, IA\"\t19171\n\"Guthrie County, IA\"\t19077\t\"Adair County, IA\"\t19001\n\"Guthrie County, IA\"\t19077\t\"Audubon County, IA\"\t19009\n\"Guthrie County, IA\"\t19077\t\"Carroll County, IA\"\t19027\n\"Guthrie County, IA\"\t19077\t\"Cass County, IA\"\t19029\n\"Guthrie County, IA\"\t19077\t\"Dallas County, IA\"\t19049\n\"Guthrie County, IA\"\t19077\t\"Greene County, IA\"\t19073\n\"Guthrie County, IA\"\t19077\t\"Guthrie County, IA\"\t19077\n\"Guthrie County, IA\"\t19077\t\"Madison County, IA\"\t19121\n\"Hamilton County, IA\"\t19079\t\"Boone County, IA\"\t19015\n\"Hamilton County, IA\"\t19079\t\"Franklin County, IA\"\t19069\n\"Hamilton County, IA\"\t19079\t\"Hamilton County, IA\"\t19079\n\"Hamilton County, IA\"\t19079\t\"Hardin County, IA\"\t19083\n\"Hamilton County, IA\"\t19079\t\"Story County, IA\"\t19169\n\"Hamilton County, IA\"\t19079\t\"Webster County, IA\"\t19187\n\"Hamilton County, IA\"\t19079\t\"Wright County, IA\"\t19197\n\"Hancock County, IA\"\t19081\t\"Cerro Gordo County, IA\"\t19033\n\"Hancock County, IA\"\t19081\t\"Franklin County, IA\"\t19069\n\"Hancock County, IA\"\t19081\t\"Hancock County, IA\"\t19081\n\"Hancock County, IA\"\t19081\t\"Humboldt County, IA\"\t19091\n\"Hancock County, IA\"\t19081\t\"Kossuth County, IA\"\t19109\n\"Hancock County, IA\"\t19081\t\"Winnebago County, IA\"\t19189\n\"Hancock County, IA\"\t19081\t\"Worth County, IA\"\t19195\n\"Hancock County, IA\"\t19081\t\"Wright County, IA\"\t19197\n\"Hardin County, IA\"\t19083\t\"Butler County, IA\"\t19023\n\"Hardin County, IA\"\t19083\t\"Franklin County, IA\"\t19069\n\"Hardin County, IA\"\t19083\t\"Grundy County, IA\"\t19075\n\"Hardin County, IA\"\t19083\t\"Hamilton County, IA\"\t19079\n\"Hardin County, IA\"\t19083\t\"Hardin County, IA\"\t19083\n\"Hardin County, IA\"\t19083\t\"Marshall County, IA\"\t19127\n\"Hardin County, IA\"\t19083\t\"Story County, IA\"\t19169\n\"Hardin County, IA\"\t19083\t\"Wright County, IA\"\t19197\n\"Harrison County, IA\"\t19085\t\"Crawford County, IA\"\t19047\n\"Harrison County, IA\"\t19085\t\"Harrison County, IA\"\t19085\n\"Harrison County, IA\"\t19085\t\"Monona County, IA\"\t19133\n\"Harrison County, IA\"\t19085\t\"Pottawattamie County, IA\"\t19155\n\"Harrison County, IA\"\t19085\t\"Shelby County, IA\"\t19165\n\"Harrison County, IA\"\t19085\t\"Burt County, NE\"\t31021\n\"Harrison County, IA\"\t19085\t\"Washington County, NE\"\t31177\n\"Henry County, IA\"\t19087\t\"Des Moines County, IA\"\t19057\n\"Henry County, IA\"\t19087\t\"Henry County, IA\"\t19087\n\"Henry County, IA\"\t19087\t\"Jefferson County, IA\"\t19101\n\"Henry County, IA\"\t19087\t\"Lee County, IA\"\t19111\n\"Henry County, IA\"\t19087\t\"Louisa County, IA\"\t19115\n\"Henry County, IA\"\t19087\t\"Van Buren County, IA\"\t19177\n\"Henry County, IA\"\t19087\t\"Washington County, IA\"\t19183\n\"Howard County, IA\"\t19089\t\"Chickasaw County, IA\"\t19037\n\"Howard County, IA\"\t19089\t\"Floyd County, IA\"\t19067\n\"Howard County, IA\"\t19089\t\"Howard County, IA\"\t19089\n\"Howard County, IA\"\t19089\t\"Mitchell County, IA\"\t19131\n\"Howard County, IA\"\t19089\t\"Winneshiek County, IA\"\t19191\n\"Howard County, IA\"\t19089\t\"Fillmore County, MN\"\t27045\n\"Howard County, IA\"\t19089\t\"Mower County, MN\"\t27099\n\"Humboldt County, IA\"\t19091\t\"Hancock County, IA\"\t19081\n\"Humboldt County, IA\"\t19091\t\"Humboldt County, IA\"\t19091\n\"Humboldt County, IA\"\t19091\t\"Kossuth County, IA\"\t19109\n\"Humboldt County, IA\"\t19091\t\"Palo Alto County, IA\"\t19147\n\"Humboldt County, IA\"\t19091\t\"Pocahontas County, IA\"\t19151\n\"Humboldt County, IA\"\t19091\t\"Webster County, IA\"\t19187\n\"Humboldt County, IA\"\t19091\t\"Wright County, IA\"\t19197\n\"Ida County, IA\"\t19093\t\"Buena Vista County, IA\"\t19021\n\"Ida County, IA\"\t19093\t\"Cherokee County, IA\"\t19035\n\"Ida County, IA\"\t19093\t\"Crawford County, IA\"\t19047\n\"Ida County, IA\"\t19093\t\"Ida County, IA\"\t19093\n\"Ida County, IA\"\t19093\t\"Monona County, IA\"\t19133\n\"Ida County, IA\"\t19093\t\"Sac County, IA\"\t19161\n\"Ida County, IA\"\t19093\t\"Woodbury County, IA\"\t19193\n\"Iowa County, IA\"\t19095\t\"Benton County, IA\"\t19011\n\"Iowa County, IA\"\t19095\t\"Iowa County, IA\"\t19095\n\"Iowa County, IA\"\t19095\t\"Johnson County, IA\"\t19103\n\"Iowa County, IA\"\t19095\t\"Keokuk County, IA\"\t19107\n\"Iowa County, IA\"\t19095\t\"Linn County, IA\"\t19113\n\"Iowa County, IA\"\t19095\t\"Poweshiek County, IA\"\t19157\n\"Iowa County, IA\"\t19095\t\"Tama County, IA\"\t19171\n\"Iowa County, IA\"\t19095\t\"Washington County, IA\"\t19183\n\"Jackson County, IA\"\t19097\t\"Carroll County, IL\"\t17015\n\"Jackson County, IA\"\t19097\t\"Jo Daviess County, IL\"\t17085\n\"Jackson County, IA\"\t19097\t\"Clinton County, IA\"\t19045\n\"Jackson County, IA\"\t19097\t\"Dubuque County, IA\"\t19061\n\"Jackson County, IA\"\t19097\t\"Jackson County, IA\"\t19097\n\"Jackson County, IA\"\t19097\t\"Jones County, IA\"\t19105\n\"Jasper County, IA\"\t19099\t\"Jasper County, IA\"\t19099\n\"Jasper County, IA\"\t19099\t\"Mahaska County, IA\"\t19123\n\"Jasper County, IA\"\t19099\t\"Marion County, IA\"\t19125\n\"Jasper County, IA\"\t19099\t\"Marshall County, IA\"\t19127\n\"Jasper County, IA\"\t19099\t\"Polk County, IA\"\t19153\n\"Jasper County, IA\"\t19099\t\"Poweshiek County, IA\"\t19157\n\"Jasper County, IA\"\t19099\t\"Story County, IA\"\t19169\n\"Jasper County, IA\"\t19099\t\"Tama County, IA\"\t19171\n\"Jefferson County, IA\"\t19101\t\"Davis County, IA\"\t19051\n\"Jefferson County, IA\"\t19101\t\"Henry County, IA\"\t19087\n\"Jefferson County, IA\"\t19101\t\"Jefferson County, IA\"\t19101\n\"Jefferson County, IA\"\t19101\t\"Keokuk County, IA\"\t19107\n\"Jefferson County, IA\"\t19101\t\"Van Buren County, IA\"\t19177\n\"Jefferson County, IA\"\t19101\t\"Wapello County, IA\"\t19179\n\"Jefferson County, IA\"\t19101\t\"Washington County, IA\"\t19183\n\"Johnson County, IA\"\t19103\t\"Benton County, IA\"\t19011\n\"Johnson County, IA\"\t19103\t\"Cedar County, IA\"\t19031\n\"Johnson County, IA\"\t19103\t\"Iowa County, IA\"\t19095\n\"Johnson County, IA\"\t19103\t\"Johnson County, IA\"\t19103\n\"Johnson County, IA\"\t19103\t\"Linn County, IA\"\t19113\n\"Johnson County, IA\"\t19103\t\"Louisa County, IA\"\t19115\n\"Johnson County, IA\"\t19103\t\"Muscatine County, IA\"\t19139\n\"Johnson County, IA\"\t19103\t\"Washington County, IA\"\t19183\n\"Jones County, IA\"\t19105\t\"Cedar County, IA\"\t19031\n\"Jones County, IA\"\t19105\t\"Clinton County, IA\"\t19045\n\"Jones County, IA\"\t19105\t\"Delaware County, IA\"\t19055\n\"Jones County, IA\"\t19105\t\"Dubuque County, IA\"\t19061\n\"Jones County, IA\"\t19105\t\"Jackson County, IA\"\t19097\n\"Jones County, IA\"\t19105\t\"Jones County, IA\"\t19105\n\"Jones County, IA\"\t19105\t\"Linn County, IA\"\t19113\n\"Keokuk County, IA\"\t19107\t\"Iowa County, IA\"\t19095\n\"Keokuk County, IA\"\t19107\t\"Jefferson County, IA\"\t19101\n\"Keokuk County, IA\"\t19107\t\"Keokuk County, IA\"\t19107\n\"Keokuk County, IA\"\t19107\t\"Mahaska County, IA\"\t19123\n\"Keokuk County, IA\"\t19107\t\"Poweshiek County, IA\"\t19157\n\"Keokuk County, IA\"\t19107\t\"Wapello County, IA\"\t19179\n\"Keokuk County, IA\"\t19107\t\"Washington County, IA\"\t19183\n\"Kossuth County, IA\"\t19109\t\"Emmet County, IA\"\t19063\n\"Kossuth County, IA\"\t19109\t\"Hancock County, IA\"\t19081\n\"Kossuth County, IA\"\t19109\t\"Humboldt County, IA\"\t19091\n\"Kossuth County, IA\"\t19109\t\"Kossuth County, IA\"\t19109\n\"Kossuth County, IA\"\t19109\t\"Palo Alto County, IA\"\t19147\n\"Kossuth County, IA\"\t19109\t\"Pocahontas County, IA\"\t19151\n\"Kossuth County, IA\"\t19109\t\"Winnebago County, IA\"\t19189\n\"Kossuth County, IA\"\t19109\t\"Wright County, IA\"\t19197\n\"Kossuth County, IA\"\t19109\t\"Faribault County, MN\"\t27043\n\"Kossuth County, IA\"\t19109\t\"Martin County, MN\"\t27091\n\"Lee County, IA\"\t19111\t\"Hancock County, IL\"\t17067\n\"Lee County, IA\"\t19111\t\"Henderson County, IL\"\t17071\n\"Lee County, IA\"\t19111\t\"Des Moines County, IA\"\t19057\n\"Lee County, IA\"\t19111\t\"Henry County, IA\"\t19087\n\"Lee County, IA\"\t19111\t\"Lee County, IA\"\t19111\n\"Lee County, IA\"\t19111\t\"Van Buren County, IA\"\t19177\n\"Lee County, IA\"\t19111\t\"Clark County, MO\"\t29045\n\"Linn County, IA\"\t19113\t\"Benton County, IA\"\t19011\n\"Linn County, IA\"\t19113\t\"Buchanan County, IA\"\t19019\n\"Linn County, IA\"\t19113\t\"Cedar County, IA\"\t19031\n\"Linn County, IA\"\t19113\t\"Delaware County, IA\"\t19055\n\"Linn County, IA\"\t19113\t\"Iowa County, IA\"\t19095\n\"Linn County, IA\"\t19113\t\"Johnson County, IA\"\t19103\n\"Linn County, IA\"\t19113\t\"Jones County, IA\"\t19105\n\"Linn County, IA\"\t19113\t\"Linn County, IA\"\t19113\n\"Louisa County, IA\"\t19115\t\"Mercer County, IL\"\t17131\n\"Louisa County, IA\"\t19115\t\"Rock Island County, IL\"\t17161\n\"Louisa County, IA\"\t19115\t\"Des Moines County, IA\"\t19057\n\"Louisa County, IA\"\t19115\t\"Henry County, IA\"\t19087\n\"Louisa County, IA\"\t19115\t\"Johnson County, IA\"\t19103\n\"Louisa County, IA\"\t19115\t\"Louisa County, IA\"\t19115\n\"Louisa County, IA\"\t19115\t\"Muscatine County, IA\"\t19139\n\"Louisa County, IA\"\t19115\t\"Washington County, IA\"\t19183\n\"Lucas County, IA\"\t19117\t\"Appanoose County, IA\"\t19007\n\"Lucas County, IA\"\t19117\t\"Clarke County, IA\"\t19039\n\"Lucas County, IA\"\t19117\t\"Decatur County, IA\"\t19053\n\"Lucas County, IA\"\t19117\t\"Lucas County, IA\"\t19117\n\"Lucas County, IA\"\t19117\t\"Marion County, IA\"\t19125\n\"Lucas County, IA\"\t19117\t\"Monroe County, IA\"\t19135\n\"Lucas County, IA\"\t19117\t\"Warren County, IA\"\t19181\n\"Lucas County, IA\"\t19117\t\"Wayne County, IA\"\t19185\n\"Lyon County, IA\"\t19119\t\"Lyon County, IA\"\t19119\n\"Lyon County, IA\"\t19119\t\"O'Brien County, IA\"\t19141\n\"Lyon County, IA\"\t19119\t\"Osceola County, IA\"\t19143\n\"Lyon County, IA\"\t19119\t\"Sioux County, IA\"\t19167\n\"Lyon County, IA\"\t19119\t\"Nobles 
